vi "Validate JWKS.vi"(8 "error in (no error)":errorcluster, 10 "kid":string, 11 "Issuer URI path":string) -> (0 "error out":errorcluster, 1 "e":string, 2 "kid found?":bool, 3 "n":string, 4 "jwks (json)":string)   [LabVIEW 2017, in "JSONWebToken.lvclass"]
doc: "Key ID (kid) is read from the JWT header and used to select from a list of known public keys.\n\nThis list is available from the host"
uses:
  JSONWebToken.lvclass
  JWKS Parameters -- cluster.ctl
  be3ffec9-44ac-4f8f-8e49-7cd159e4ab34.vi
  61810052-8a2d-4f14-a566-0ae808cfdb65.vi
  <vilib>/JDP Science/JSONtext/Find Item.vi
  <vilib>/JDP Science/JSONtext/Find Multiple Items.vi
  <vilib>/JDP Science/JSONtext/Next JSON Value.vi
  <vilib>/JDP Science/JSONtext/String Subset.vi
  <vilib>/JDP Science/JSONtext/support/Strip Quotes and Unescape.vi
  <vilib>/JDP Science/JSONtext/Parsing/Advance past next JSON Value (inlined COPY).vi
  <vilib>/JDP Science/JSONtext/support/Unescape JSON string.vi
  <vilib>/JDP Science/JSONtext/Parsing/Advance past whitespace.vi
  <vilib>/JDP Science/JSONtext/Parsing/Advance past String.vi
  <vilib>/JDP Science/JSONtext/Parsing/Advance past Number.vi
  <vilib>/JDP Science/JSONtext/Parsing/Advance past Line Ending.vi
  <vilib>/JDP Science/JSONtext/Parsing/Parse Full Path or Item Name.vi
  <vilib>/JDP Science/JSONtext/Parsing/Advance past Array.vi
  <vilib>/JDP Science/JSONtext/Parsing/Advance past Object.vi
  <vilib>/JDP Science/JSONtext/support/Error Cluster From Code.vi
  <vilib>/JDP Science/JSONtext/Offset/Find Item Locations by Path.vi
  <vilib>/JDP Science/JSONtext/JSON text to Variant.vi
  <vilib>/JDP Science/JSONtext/LVClass Serializer/JSONtext LVClass Serializer.lvclass
  <vilib>/httpClient/LabVIEWHTTPClient.lvlib
  <vilib>/LabVIEW Open Source Project/OpenSerializer.Base64/Serializer.Base64.lvclass
panel:
  # "https://openid.net/specs/openid-connect-basic-1_0.html#IDTokenValidation"
  # "https://dev.to/kimmaida/signing-and-validating-json-web-tokens-jwt-for-everyone-25fb"
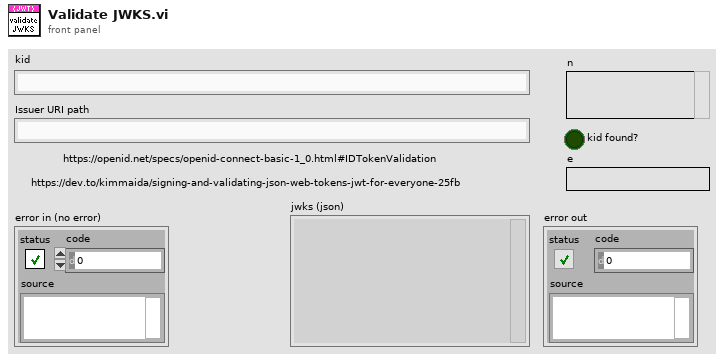
[diagram p1: front panel]
types:
  T1 = typedef "JSONWebToken.lvclass/JWKS Parameters -- cluster.ctl" = cluster{"kty":string, "use":string, "kid":string, "alg":string, "n":string, "e":string, "k":string, "x":string, "y":string, "crv":string, "key_ops":string}
  T2 = typedef "LabVIEWHTTPClient.lvlib/ClientHandle.ctl" = refnum<k1>
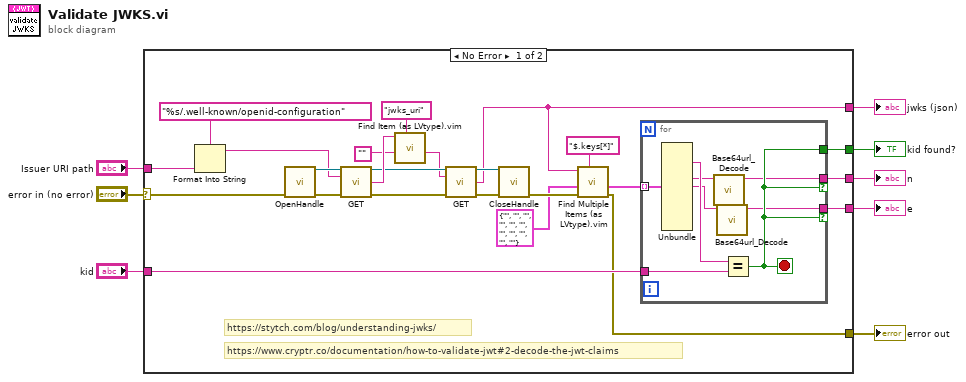
[diagram p0: block diagram]
diagram:
  n1 = case shown="No Error" "error in (no error)" {
    selector: "error in (no error)" -> [w16 w41]
    tunnel: "Issuer URI path" -> [w10 _]
    tunnel: "kid" -> [w23 _]
    tunnel: [w22 _] -> w6
    tunnel: [w21 _] -> w5
    tunnel: [w17 w41] -> w4
    tunnel: [w13 _] -> w2
    tunnel: [w15 _] -> w1
    frame No Error {
      # "https://www.cryptr.co/documentation/how-to-validate-jwt#2-decode-the-jwt-claims"
      # "https://stytch.com/blog/understanding-jwks/"
      n2 = Format Into String(format string="%s/.well-known/openid-configuration" ("url"), w10) -> (resulting string=w9:string)  [unwired: 2 in, 1 out]
      n3 = call <vilib>:"OpenHandle.vi"("error in (no error)"=w16) -> ("client handle out"=w32:T2, "error out"=w31:errorcluster)  [unwired: 13 in]
      n4 = call <vilib>:"GET.vi"("client handle"=w32, "url"=w9, "error in (no error)"=w31) -> ("client handle out"=w28:T2, "body"=w30:string, "error out"=w27:errorcluster)  [unwired: 9 in, 1 out]
      n5 = call "Find Item (as LVtype).vim"("$Path or Item Name"="jwks_uri", "Data Type and Default Value"="", "JSON"=w30) -> ("Data"=w20:string)  [unwired: 5 in, 3 out]
      n6 = call <vilib>:"GET.vi"("client handle"=w28, "url"=w20, "error in (no error)"=w27) -> ("client handle out"=w25:T2, "body"=w13:string, "error out"=w26:errorcluster)  [unwired: 9 in, 1 out]
      n7 = call <vilib>:"CloseHandle.vi"("client handle"=w25, "error in (no error)"=w26) -> ("error out"=w19:errorcluster)  [unwired: 13 in]
      n8 = call "Find Multiple Items (as LVtype).vim"("$Path or Item Name"="$.keys[*]", "error in (no error)"=w19, "Data Type and Default Value"=T1 {"kty"="", "use"="", "kid"="", "alg"="", "n"="", "e"="", "k"="", "x"="", "y"="", "crv"="", "key_ops"=""} ("jwks"), "JSON"=w13) -> ("error out"=w17:errorcluster, "Array of Data"=w12:T1[])  [unwired: 4 in, 2 out]
      n9 = for {
        tunnel: w12 -> [w40] mode=indexing
        tunnel: w23 -> [w38]
        tunnel: [w34] -> w22 if=w37
        tunnel: [w33] -> w15 if=w37
        tunnel: [w37] -> w21
        stop <- w37 stop-if-true
        n10 = Unbundle(w40) -> ("kid"=w39:string, "n"=w36:string, "e"=w35:string)  [unwired: 8 out]
        n11 = call <vilib>:"Base64url_Decode.vi"("Base64 URL String"=w36) -> ("Decoded String"=w34:string)  [unwired: 9 in, 1 out]
        n12 = call <vilib>:"Base64url_Decode.vi"("Base64 URL String"=w35) -> ("Decoded String"=w33:string)  [unwired: 9 in, 1 out]
        n13 = Equal?(x=w39, y=w38) -> (x = y?=w37:bool)
      }
    }
    frame Error {
    }
  }
  "n" <- w6
  "e" <- w1
  "kid found?" <- w5
  "error out" <- w4
  "jwks (json)" <- w2
